vi "add assembly.vi"(4 "data type":T1, 5 "big endian?":bool, 6 "size (elements)":u32=4, 7 "name":string, 8 "error in":errorcluster, 9 "Type":T2, 10 "instance ID":u32=100, 11 "EthernetIP configuration in":refnum<class "EthernetIP configuration.lvclass">) -> (0 "error out":errorcluster, 3 "EthernetIP configuration out":refnum<class "EthernetIP configuration.lvclass">)   [LabVIEW 2013, in "EthernetIP configuration.lvclass"]
uses:
  EthernetIP configuration.lvclass
  assembly type.ctl
  <vilib>/NI/Tag Bus/tag/Data Type.ctl
  EthernetIP configuration.lvclass/EthernetIP configuration.ctl
  assembly definition.ctl
  <vilib>/NI/Tag Bus/tag/tag descriptor.lvclass
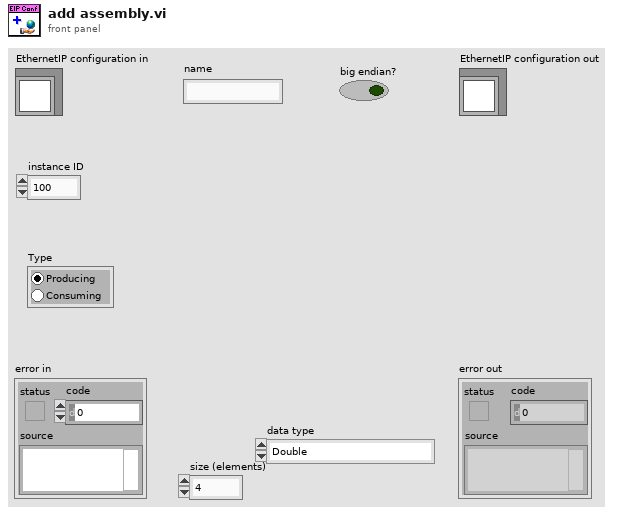
[diagram p1: front panel]
types:
  T1 = typedef "tag bus.lvlib/tag descriptor.lvclass/Data Type.ctl" = enum16{"Double", "Single", "I64", "I32", "I16", "I8", "U64", "U32", "U16", "U8", "Boolean", "String", "Array of Double", "Array of Single", "Array of I64", "Array of I32", "Array of I16", "Array of I8", "Array of U64", "Array of U32", "Array of U16", "Array of U8", "Array of Boolean", "Array of String"}
  T2 = typedef "EthernetIP configuration.lvclass/assembly type.ctl" = enum32{"Producing", "Consuming"}
  T3 = typedef "EthernetIP configuration.lvclass/assembly definition.ctl" = cluster{"name":string, "Instance ID":u32, "Type":T2, "Size (elements)":u32, "big endian?":bool, "data type":T1}
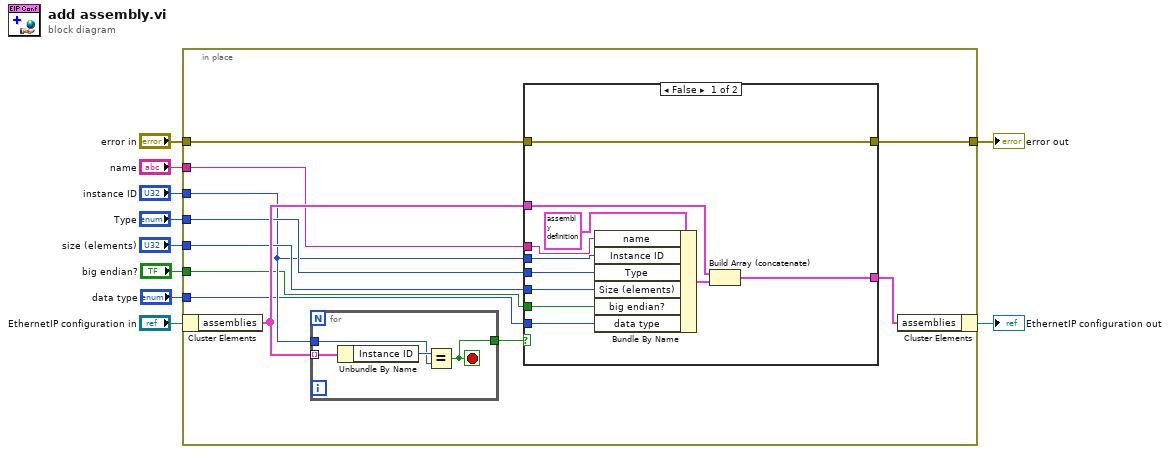
[diagram p0: block diagram]
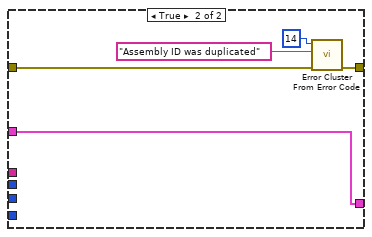
[diagram p2: hidden frame]
diagram:
  n1 = in-place {
    in-place-border: "instance ID" -> [w14]
    in-place-border: "error in" -> [w18]
    in-place-border: [w17] -> w6
    in-place-border: "size (elements)" -> [w16]
    in-place-border: "Type" -> [w15]
    in-place-border: "name" -> [w13]
    in-place-border: "big endian?" -> [w12]
    in-place-border: "data type" -> [w11]
    n2 = in-place-cluster #1("EthernetIP configuration in") -> ("assemblies"=w19:T3[])
    n3 = for {
      tunnel: w19 -> [w41] mode=indexing
      tunnel: w14 -> [w39]
      tunnel: [w38] -> w21
      stop <- w38 stop-if-true
      n4 = Unbundle By Name(w41) -> ("Instance ID"=w40:u32)
      n5 = Equal?(x=w40, y=w39) -> (x = y?=w38:bool)
    }
    n6 = case shown="False" w21 {
      tunnel: [w30 w37] -> w20
      tunnel: w19 -> [w31 w37]
      tunnel: w18 -> [w32 w34]
      tunnel: [w32 w33] -> w17
      tunnel: w16 -> [w28 _]
      tunnel: w15 -> [w27 _]
      tunnel: w14 -> [w26 _]
      tunnel: w13 -> [w25 _]
      tunnel: w12 -> [w23 _]
      tunnel: w11 -> [w22 _]
      frame False {
        n7 = Bundle By Name(cluster=T3 {"name"="", "Instance ID"=100, "Type"=enum."Producing", "Size (elements)"=32, "big endian?"=FALSE, "data type"=enum."Double"} ("assembly definition"), "name"=w25, "Instance ID"=w26, "Type"=w27, "Size (elements)"=w28, "big endian?"=w23, "data type"=w22) -> (w24:T3)
        n8 = Build Array (concatenate)(w31, w24) -> (w30:T3[])
      }
      frame True {
        n9 = call <vilib>:"Error Cluster From Error Code.vi"("error in (no error)"=w34, "error message (\"\")"="Assembly ID was duplicated" ("error message (\"\")"), "error code (0)"=14) -> ("error out"=w33:errorcluster)  [unwired: 6 in]
      }
    }
    n10 = in-place-cluster #1("assemblies"=w20) -> (→"EthernetIP configuration out":refnum<class "EthernetIP configuration.lvclass">)
  }
  "error out" <- w6
